vi "2D DST.vi"(11 "X":dbl[][](array[numeric])) -> (0 "error":i32, 3 "DST {X}":dbl[][](array[numeric]))   [LabVIEW 2018, in "NI_AALPro.lvlib"]
doc: "Computes the Discrete Sine Transform (DST) of the input sequence <B>X</B>. Wire data to the <B>X</B> input to determine the polymorphic instance to use or manually select the instance."
uses:
  NI_AALPro.lvlib
  <resource>/lvanlys.dll
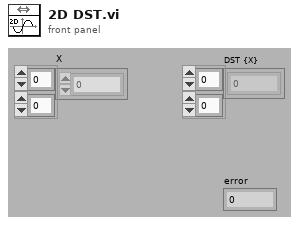
[diagram p1: front panel]
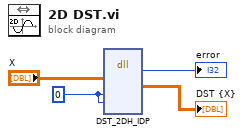
[diagram p0: block diagram]
diagram:
  w1 = 0 ("rows")
  n1 = dll-call lib="C:/Program Files (x86)/National Instruments/LabVIEW 2018/resource/lvanlys.*" fn="DST_2DH_IDP"("xH"="X", "rows"=w1, "cols"=w1) -> ("return type"=→"error":i32, "yH"=→"DST {X}":dbl[][])  [unwired: 9 in, 2 out]
